vi "FGV Gasteilerliste laden.vi"(6 "Aktion":T2, 8 "error in (no error)":errorcluster caption="Fehler (Eingang, kein Fehler)", 10 "PrüfgasName":T1 caption="Formula:", 11 "Gasindex":i32) -> (0 "error out":errorcluster caption="Fehler (Ausgang)", 2 "Formel":string, 3 "Summenformeln":string[](array[string]))   [LabVIEW 2020, in "Linearisierung v2.lvlib" / "Gasteiler.lvlib"]
uses:
  Gasteiler.lvlib
  Aktion FGV Gasteilerliste laden.ctl
  Visualisierungs Elemente/String - Eingabefeld.ctl
  SummenformelCluster.ctl
  Seiten/FT-IR/FGV FT-IR Gasliste Aktionen.ctl
  Allgemein/allgemeine Sub-VIs.lvlib
  Seiten/Gaszuordnung AO/Gaszuordnung AO.lvlib
  Seiten/FT-IR/FT-IR.lvlib
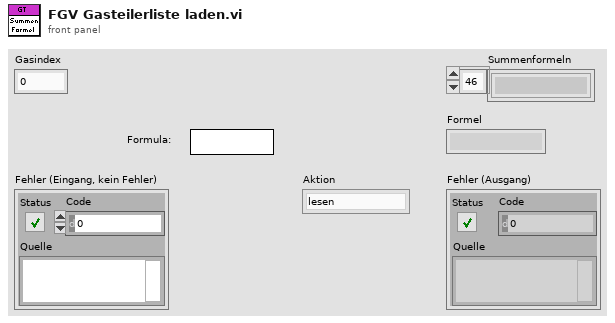
[diagram p1: front panel]
types:
  T1 = typedef "String - Eingabefeld.ctl" = string
  T2 = typedef "Linearisierung v2.lvlib/Gasteiler.lvlib/Aktion FGV Gasteilerliste laden.ctl" = enum16{"lesen", "laden", "speichern", "Liste erstellen", "Formel ändern", "Gas vereinzeln"}
  T3 = typedef "Linearisierung v2.lvlib/Gasteiler.lvlib/SummenformelCluster.ctl" = cluster{"Gasnamen":string[], "Summenformel":string[]}
  T4 = typedef "FT-IR.lvlib/FGV FT-IR Gasliste Aktionen.ctl" = enum16{"lesen", "Gasliste FT-IR", "Gasliste ausgelesen", "laden", "speichern", "löschen"}
  T5 = typedef "String - Ausgabefeld.ctl" = string
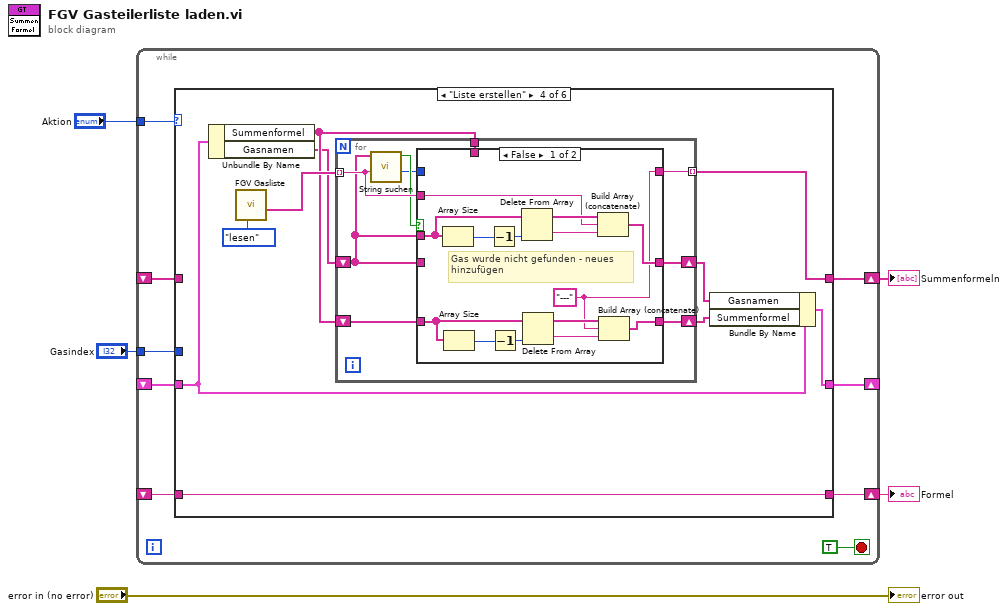
[diagram p0: block diagram]
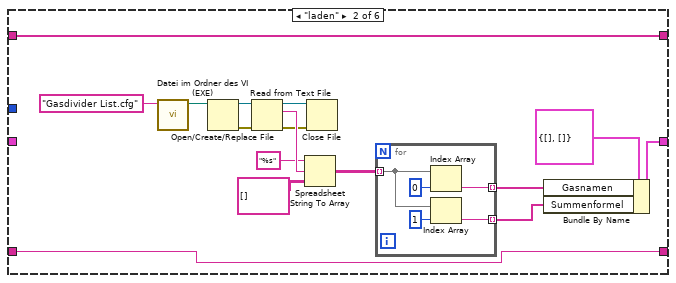
[diagram p3: hidden frame]
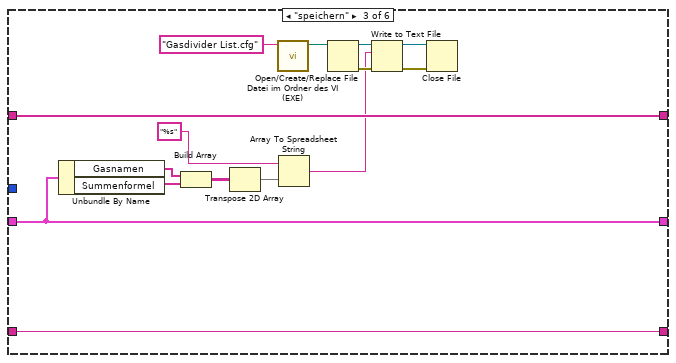
[diagram p4: hidden frame]
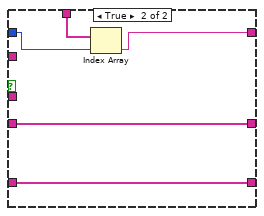
[diagram p5: hidden frame]
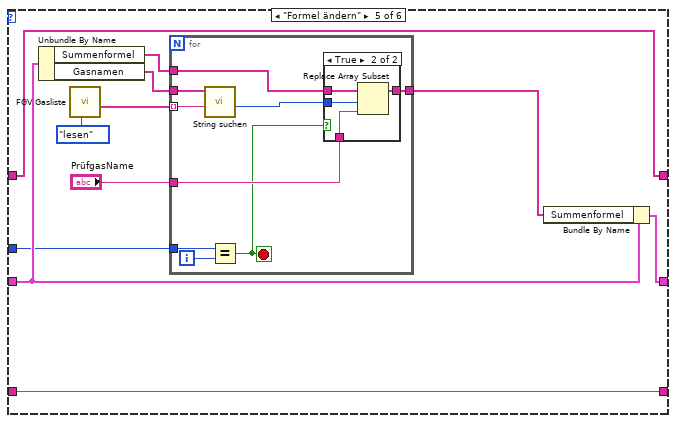
[diagram p6: hidden frame]
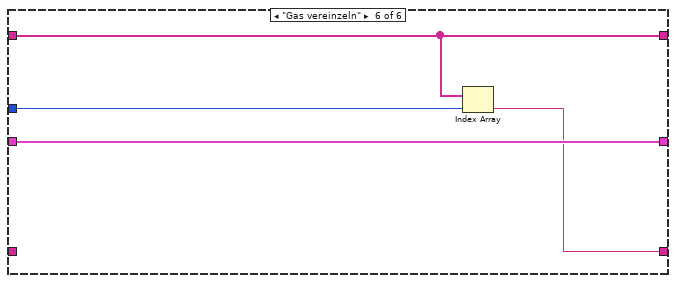
[diagram p8: hidden frame]
diagram:
  n1 = while {
    tunnel: "Aktion" -> [w14]
    shift-right: [w12] -> _
    shift-left: _ -> [w11]
    shift-right: [w10] -> w4
    shift-left: _ -> [w9]
    tunnel: "Gasindex" -> [w8]
    shift-right: [w7] -> w2
    shift-left: _ -> [w6]
    stop <- TRUE stop-if-true
    n2 = case shown="\"Liste erstellen\"" w14 {
      tunnel: [w17 w20 w45 w56 w97 w120] -> w12
      tunnel: w11 -> [w17 _ w45 w57 w98 w120]
      tunnel: [w16 w19 w53 w63 w92 w119] -> w10
      tunnel: w9 -> [w16 w19 w53 _ w92 w119]
      tunnel: w8 -> [_ _ _ _ w96 w118]
      tunnel: [w15 w18 w52 w60 w100 w117] -> w7
      tunnel: w6 -> [w15 w18 w52 w60 w100 _]
      frame "lesen", Default {
      }
      frame "laden" {
        n3 = call "Datei im Ordner des VI (EXE).vi"("Dateiname"="Gasdivider List.cfg") -> ("Dateipfad im Ordner des Haupt-VIs"=w26:path)  [unwired: 8 in, 2 out]
        n4 = Open/Create/Replace File(file path (use dialog)=w26) -> (refnum out=w28:refnum<file>, error out=w27:errorcluster)  [unwired: 1 in, 5 out]
        n5 = Read from Text File(file (use dialog)=w28, error in=w27) -> (refnum out=w30:refnum<file>, text=w33:string, error out=w29:errorcluster)  [unwired: 3 out]
        n6 = Spreadsheet String To Array(format string="%s" ("Format-String"), spreadsheet string=w33, array type (2D Dbl)=string[][] []) -> (array=w21:string[][])  [unwired: 1 out]
        n7 = Close File(refnum=w30, error in=w29) -> ()  [unwired: 2 out]
        n8 = for {
          tunnel: w21 -> [w34] mode=indexing
          tunnel: [w36] -> w23 mode=indexing
          tunnel: [w35] -> w24 mode=indexing
          n9 = Index Array(array=w34, index=0 ("Index")) -> (element=w36:string)
          n10 = Index Array(array=w34, index=1 ("Index")) -> (element=w35:string)
        }
        n11 = Bundle By Name(cluster=T3 {"Gasnamen"=[], "Summenformel"=[]} ("Polynome"), "Gasnamen"=w23, "Summenformel"=w24) -> (w20:T3)
      }
      frame "speichern" {
        n12 = Unbundle By Name(w45) -> ("Gasnamen"=w44:string[], "Summenformel"=w43:string[])
        n13 = Build Array(w44, w43) -> (w40:string[][])
        n14 = Transpose 2D Array(2D array=w40) -> (transposed array=w39:string[][])
        n15 = call "Datei im Ordner des VI (EXE).vi"("Dateiname"="Gasdivider List.cfg") -> ("Dateipfad im Ordner des Haupt-VIs"=w47:path)  [unwired: 8 in, 2 out]
        n16 = Array To Spreadsheet String(array=w39, 3:"%s" ("Format-String")) -> (spreadsheet string=w41:string)  [unwired: 1 in]
        n17 = Open/Create/Replace File(file path (use dialog)=w47) -> (refnum out=w49:refnum<file>, error out=w48:errorcluster)  [unwired: 1 in, 5 out]
        n18 = Write to Text File(file (use dialog)=w49, text=w41, error in=w48) -> (refnum out=w51:refnum<file>, error out=w50:errorcluster)  [unwired: 1 in, 1 out]
        n19 = Close File(refnum=w51, error in=w50) -> ()  [unwired: 2 out]
      }
      frame "Liste erstellen" {
        n20 = Unbundle By Name(w57) -> ("Summenformel"=w59:string[], "Gasnamen"=w58:string[])
        n21 = call "FGV Gasliste.vi"("Aktionen"=FGV_FT-IR_Gasliste_Aktionen."lesen") -> ("Aktuelle Gasliste gesamt"=w61:T5[])  [unwired: 8 in, 2 out]
        n22 = for {
          tunnel: w61 -> [w72] mode=indexing
          tunnel: w59 -> [w66]
          tunnel: [w65] -> w63 mode=indexing
          shift-right: [w70] -> w55
          shift-left: w58 -> [w67]
          shift-right: [w68] -> w54
          shift-left: w59 -> [w69]
          n23 = call "String suchen.vi"("Gasname"=w72, "Such-Namen"=w67) -> ("Index"=w64:i32, "Gefunden?"=w71:bool)  [unwired: 8 in]
          n24 = case shown="False" w71 {
            tunnel: w67 -> [w86 _]
            tunnel: w72 -> [w82 _]
            tunnel: [w80 w91] -> w70
            tunnel: w67 -> [_ w91]
            tunnel: w69 -> [w75 w90]
            tunnel: [w74 w90] -> w68
            tunnel: w66 -> [_ w89]
            tunnel: [w73 w88] -> w65
            tunnel: w64 -> [_ w87]
            frame False {
              w73 = "---" ("Element")
              # "Gas wurde nicht gefunden - neues\nhinzufügen"
              n25 = Array Size(array=w86) -> (size(s)=w85:i32)
              n26 = Array Size(array=w75) -> (size(s)=w76:i32)
              n27 = Decrement(x=w85) -> (x-1=w84:i32)
              n28 = Decrement(x=w76) -> (x-1=w77:i32)
              n29 = Delete From Array(array=w86, index=w84) -> (deleted portion=w81:T5, array with subset deleted=w83:T5[])  [unwired: 1 in]
              n30 = Delete From Array(array=w75, index=w77) -> (deleted portion=w79:string, array with subset deleted=w78:string[])  [unwired: 1 in]
              n31 = Build Array (concatenate)(w83, w82, w81) -> (w80:T5[])
              n32 = Build Array (concatenate)(w78, w73, w79) -> (w74:string[])
            }
            frame True {
              n33 = Index Array(array=w89, index=w87) -> (element=w88:string)
            }
          }
        }
        n34 = Bundle By Name(cluster=w57, "Gasnamen"=w55, "Summenformel"=w54) -> (w56:T3)
      }
      frame "Formel ändern" {
        n35 = Unbundle By Name(w98) -> ("Summenformel"=w93:string[], "Gasnamen"=w99:string[])
        n36 = call "FGV Gasliste.vi"("Aktionen"=FGV_FT-IR_Gasliste_Aktionen."lesen") -> ("Aktuelle Gasliste gesamt"=w101:T5[])  [unwired: 8 in, 2 out]
        n37 = for {
          tunnel: w101 -> [w110] mode=indexing
          tunnel: w99 -> [w111]
          tunnel: w93 -> [w107]
          tunnel: w96 -> [w108]
          tunnel: [w106] -> w94
          tunnel: "PrüfgasName" -> [w104]
          i -> [w109]
          stop <- w103 stop-if-true
          n38 = call "String suchen.vi"("Gasname"=w110, "Such-Namen"=w111) -> ("Index"=w105:i32)  [unwired: 8 in, 1 out]
          n39 = Equal?(x=w108, y=w109) -> (x = y?=w103:bool)
          n40 = case shown="True" w103 {
            tunnel: w107 -> [w112 w116]
            tunnel: [w112 w115] -> w106
            tunnel: w105 -> [_ w114]
            tunnel: w104 -> [_ w113]
            frame False {
            }
            frame True {
              n41 = Replace Array Subset(array=w116, new element=w113, index=w114) -> (w115:string[])
            }
          }
        }
        n42 = Bundle By Name(cluster=w98, "Summenformel"=w94) -> (w97:T3)
      }
      frame "Gas vereinzeln" {
        n43 = Index Array(array=w119, index=w118) -> (element=w117:string)
      }
    }
  }
  "Summenformeln" <- w4
  "Formel" <- w2
  "error out" <- "error in (no error)"
